vi "Test_Encoders.vi"() -> ()   [LabVIEW 2014]
uses:
  <userlib>/UCSD Robotics Lab/Robotics-Cape/LV/libroboticscape.lvlib
panel:
  out "Timing Block":T1 {"Actual Hz" format="%#_3g"; "Dt" format="%#_4g"; "Average Hz" format="%#_4g"}
  in  "Channel":T2(ring)=enum."Encoder 2"
  in  "value":i32
  in  "Reset Encoders":bool
  in  "Set Encoder":bool
  out "Encoder Data":T3
  out "State":T4(ring)
  in  "stop":bool
  # "Always stop the VI using the rectangular STOP button above, never with the round stopsign (Abort)"
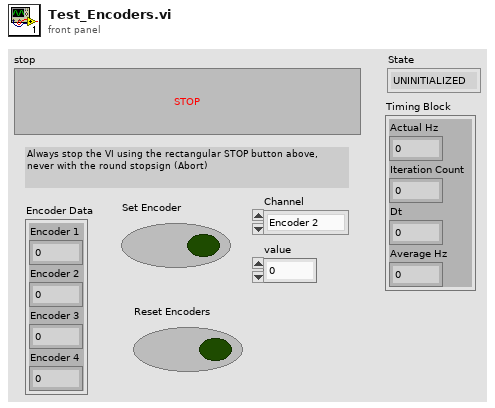
[diagram p1: front panel]
types:
  T1 = cluster{"Actual Hz":dbl, "Iteration Count":dbl, "Dt":dbl, "Average Hz":dbl}
  T2 = enum16{"", "Encoder 1", "Encoder 2", "Encoder 3", "Encoder 4"}
  T3 = cluster{"Encoder 1":i32, "Encoder 2":i32, "Encoder 3":i32, "Encoder 4":i32}
  T4 = enum16{"UNINITIALIZED", "RUNNING", "PAUSED", "EXITING"}
  T5 = enum16{"UNINITIALIZED", "RUNING", "PAUSED", "EXITING"}
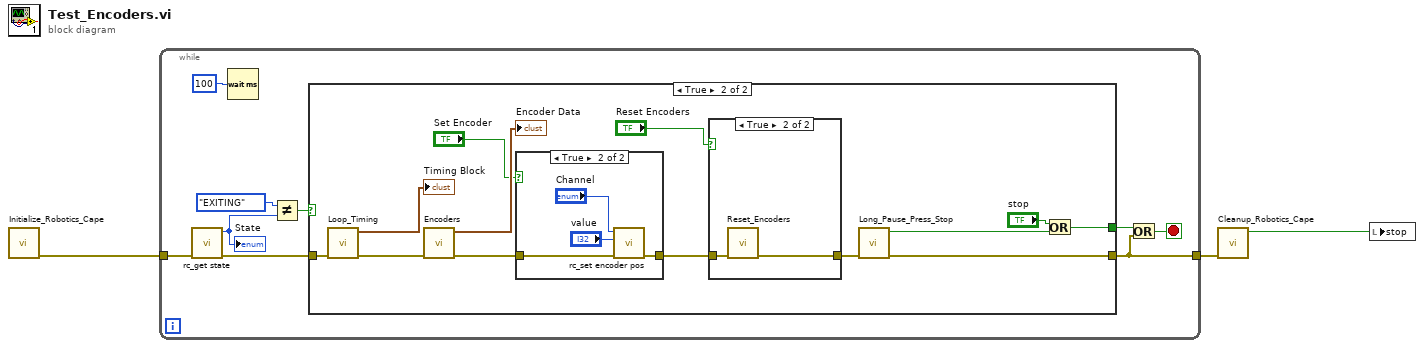
[diagram p0: block diagram]
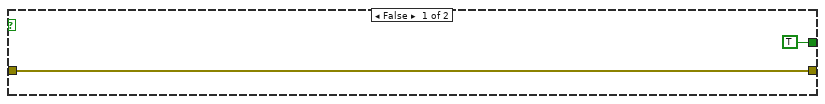
[diagram p2: hidden frame]
diagram:
  n1 = call "Initialize_Robotics_Cape.vi"() -> ("error out"=w3:errorcluster)  [unwired: 11 in]
  n2 = while {
    tunnel: w3 -> [w11]
    tunnel: [w5] -> w2
    stop <- w12 stop-if-true
    n3 = call <userlib>:"rc_get state.vi"("error in (no error)"=w11) -> ("error out"=w10:errorcluster, "function return"=w9:u32)  [unwired: 9 in]
    "State" <- w9
    n4 = Wait (ms)(milliseconds to wait=u32 100) -> ()  [unwired: 1 out]
    n5 = Not Equal?(x=T5."EXITING" ("State 2"), y=w9) -> (x != y?=w8:bool)
    n6 = case shown="True" w8 {
      tunnel: w10 -> [w14 w22]
      tunnel: [w14 w15] -> w5
      tunnel: [TRUE ("stop") w18] -> w6
      frame False {
      }
      frame True {
        n7 = call "Loop_Timing.vi"("error in"=w22) -> ("error out"=w21:errorcluster, "Timing Block"=→"Timing Block":T1)  [unwired: 9 in]
        n8 = call "Encoders.vi"("error in (no error)"=w21) -> ("error out"=w23:errorcluster, "Encoder Data"=→"Encoder Data":T3)  [unwired: 9 in]
        n9 = case shown="True" "Set Encoder" {
          tunnel: w23 -> [w31 w35]
          tunnel: [w31 w34] -> w24
          frame False {
          }
          frame True {
            n10 = call <userlib>:"rc_set encoder pos.vi"("error in (no error)"=w35, "value"="value", "ch"="Channel") -> ("error out"=w34:errorcluster)  [unwired: 7 in, 1 out]
          }
        }
        n11 = case shown="True" "Reset Encoders" {
          tunnel: w24 -> [w28 w30]
          tunnel: [w28 w29] -> w16
          frame False {
          }
          frame True {
            n12 = call "Reset_Encoders.vi"("error in (no error)"=w30) -> ("error out"=w29:errorcluster)  [unwired: 10 in]
          }
        }
        n13 = call "Long_Pause_Press_Stop.vi"("error in (no error)"=w16) -> ("error out"=w15:errorcluster, "Stop"=w17:bool)  [unwired: 9 in]
        n14 = Or(x="stop", y=w17) -> (x .or. y?=w18:bool)
      }
    }
    n15 = Or(x=w6, y=w5) -> (x .or. y?=w12:bool)
  }
  n16 = call "Cleanup_Robotics_Cape.vi"("error in (no error)"=w2) -> ("Stop Local Variabl"=w1:bool)  [unwired: 9 in, 1 out]
  n17 = local write "stop"(w1) -> ()
